vi "S71200_PLC_2.vi"(11 "Simulazione":bool) -> ()   [LabVIEW 2019]
uses:
  Uscite PLC 2.ctl
  controls/statoAO_plc_2.ctl
  StatoDO_PLC_2.ctl
  STATO PLC 2.ctl
  TypeDef_PLC_Q.ctl
  TypeDef/DEVICE NAME.ctl
  STATO PLC 1.ctl
  Uscite PLC 1.ctl
  controls/statoAO_plc_1.ctl
  StatoDO_PLC_1.ctl
  SIEMENS/S7Com_Source/S7Com_RW_CMD.ctl
  SIEMENS/S7Com_Source/S7Com_Address_Area.ctl
  SIEMENS/S7Com_Source/S7Com_Start_Add.ctl
  SIEMENS/S7Com_Source/S7Com_Transport_Size.ctl
  SIEMENS/S7Com_Source/S7Com_Function.ctl
panel:
  in  "millisecond multiple":u32=100
  out "write ao":errorcluster
  out "initialize":errorcluster
  in  "Tab Control":enum32{"PLC", "MERKER ", "DATABLOCK", "FGD"}(tab)
  out "STATO PLC":T1
  in  "write":bool
  in  "USCITE PLC":T2
  out "IP":string
  out "Simulazione 2":bool
  out "# elements in queue":i32
  out "DESC SCRITTURE MERKER WORD (AO)":string[][](array[string])
  out "Array WORD out":dbl[](array[numeric])
  out "DESC LETTURE MERKER WORD (AI)":string[][](array[string])
  out "MW read":dbl[](array[numeric])
  out "DESC SCRITTURE MERKER BIT (DO)":string[][](array[string])
  out "stato uscite DO":bool[](array[boolean])
  out "DESC LETTURE MERKER BIT (DI)":string[][](array[string])
  out "MBit read":bool[](array[boolean])
  out "DESC SCRITTURE MERKER REAK (AO)":string[][](array[string])
  out "DESC LETTURE MERKER REAL (AI)":string[][](array[string])
  out "Array M REAL out":dbl[](array[numeric])
  out "M Real":dbl[](array[numeric]) format="%.5f"
  out "DESC SCRITTURE DB BIT (DO)":string[][](array[string])
  out "DESC LETTURE DB BIT (DI)":string[][](array[string])
  out "DESC SCRITTURE DB WORD (AO)":string[][](array[string])
  out "DESC LETTURE DB WORD (AI)":string[][](array[string])
  out "DESC LETTURE DB REAL (AI)":string[][](array[string])
  out "DESC SCRITTURE DB REAL (AO)":string[][](array[string])
  out "DB WORD":dbl[](array[numeric])
  out "DB REAL":dbl[](array[numeric]) format="%.6f"
  out "Array DB bit":bool[](array[boolean])
  out "Array DB W out":dbl[](array[numeric])
  out "Array DB REAL out":dbl[](array[numeric]) format="%#.5f"
  out "DO (DATABLOCK)":bool[](array[boolean])
  out "M BIT SCRITTURE":cluster{"M":i16, "BIT":i16[]}[](array[cluster])
  out "M BIT LETTURE":cluster{"M":i16, "BIT":i16[]}[](array[cluster])
  out "MW SCRITTURE":T5(array[cluster])
  out "MW LETTURE":T5(array[cluster])
  out "M REAL LETTURE":cluster{"MD":i16, "Descrizione":string}[](array[cluster])
  out "M REAL SCRITTURE (AO)":cluster{"MD":i16, "Descrizione":string}[](array[cluster])
  out "DBW LETTURE":T6(array[cluster])
  out "DB REAL LETTURE":T7(array[cluster])
  out "DBW SCRITTURE":T6(array[cluster])
  out "DB REAL SCRITTURE":T7(array[cluster])
  out "DB BIT LETTURE":cluster{"DB":i16, "BIT":i16[], "DBoffset":i16}[](array[cluster])
  out "DB BIT SCRITTURE":cluster{"DB":i16, "BIT":i16[], "DBoffset":i16}[](array[cluster])
  out "Message":string
  out "write do":errorcluster
  out "read":errorcluster
  out "error out":errorcluster
  out "Numeric":i32
  out "Tread ms":u32
  in  "stop":bool
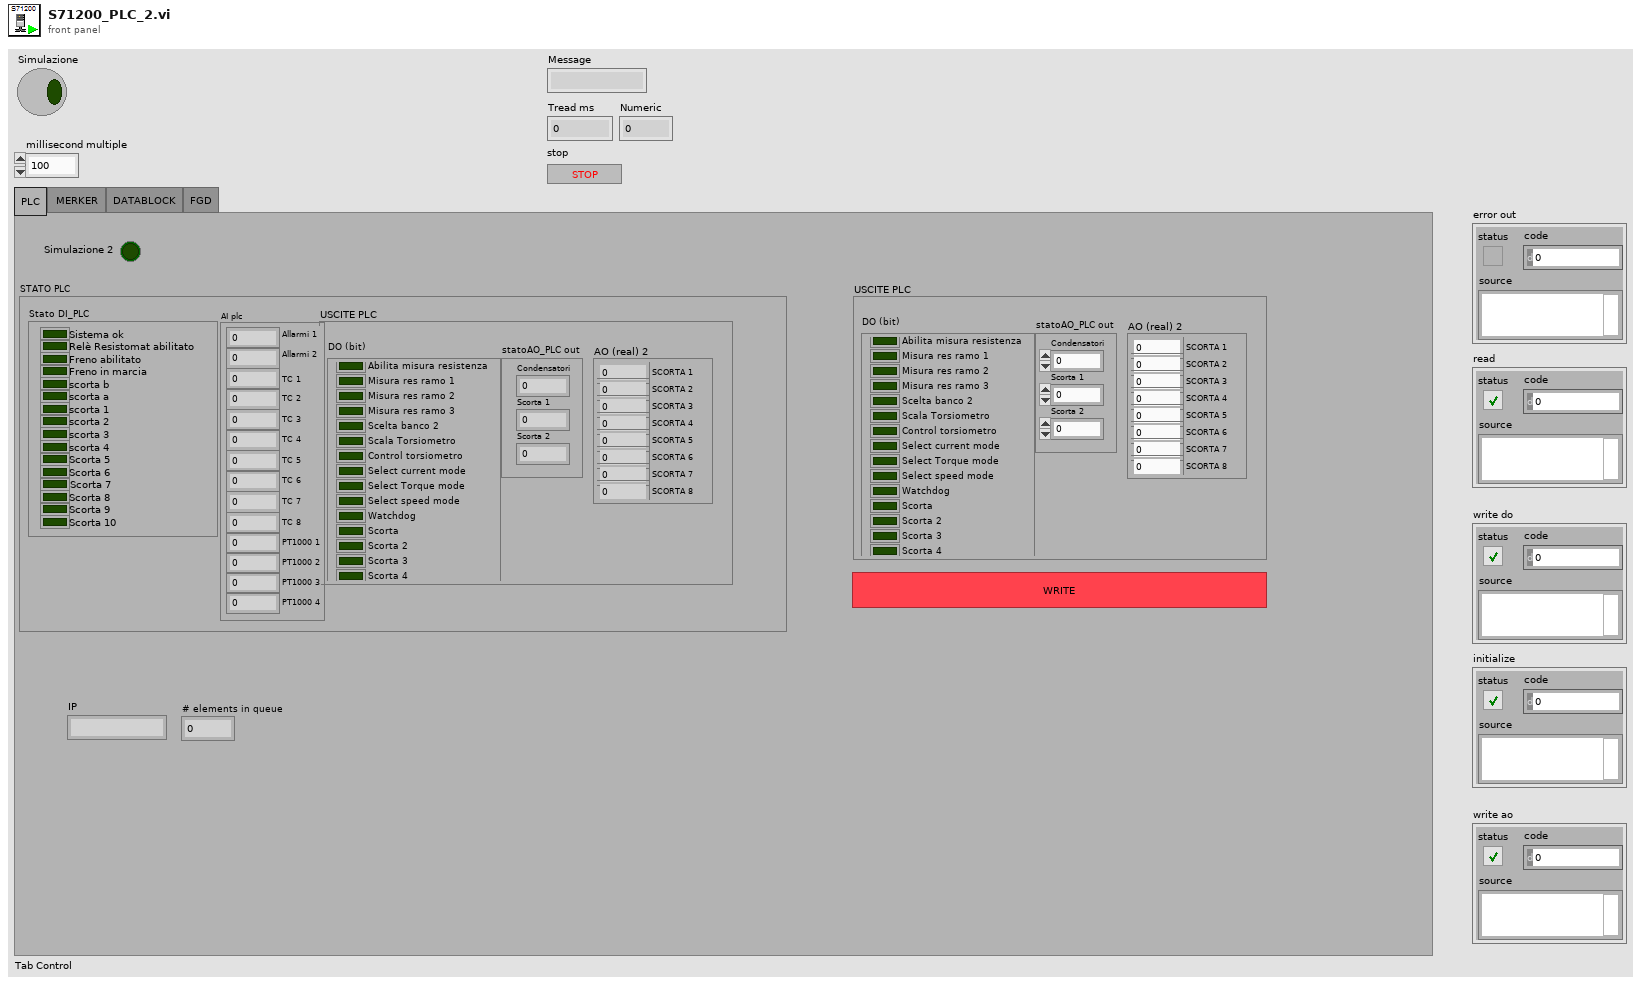
[diagram p1: front panel]
types:
  T1 = typedef "STATO PLC 2.ctl" = cluster{"USCITE PLC":T2, "Stato DI_PLC":cluster{"Sistema ok":bool, "Relè Resistomat abilitato":bool, "Freno abilitato":bool, "Freno in marcia":bool, "scorta b":bool, "scorta a":bool, "scorta 1":bool, "scorta 2":bool, "scorta 3":bool, "scorta 4":bool, "Scorta 5":bool, "Scorta 6":bool, "Scorta 7":bool, "Scorta 8":bool, "Scorta 9":bool, "Scorta 10":bool}, "AI plc":cluster{"Allarmi 1":dbl, "Allarmi 2":dbl, "TC 1":dbl, "TC 2":dbl, "TC 3":dbl, "TC 4":dbl, "TC 5":dbl, "TC 6":dbl, "TC 7":dbl, "TC 8":dbl, "PT1000 1":dbl, "PT1000 2":dbl, "PT1000 3":dbl, "PT1000 4":dbl}}
  T2 = typedef "Uscite PLC 2.ctl" = cluster{"AO (real) 2":cluster{"SCORTA 1":dbl, "SCORTA 2":dbl, "SCORTA 3":dbl, "SCORTA 4":dbl, "SCORTA 5":dbl, "SCORTA 6":dbl, "SCORTA 7":dbl, "SCORTA 8":dbl}, "statoAO_PLC out":T3, "DO (bit)":T4}
  T3 = typedef "statoAO_plc_2.ctl" = cluster{"Condensatori":dbl, "Scorta 1":dbl, "Scorta 2":dbl}
  T4 = typedef "StatoDO_PLC_2.ctl" = cluster{"Relè misura resistomat":bool, "Misura res ramo 1":bool, "Misura res ramo 2":bool, "Misura res ramo 3":bool, "Scelta banco 2":bool, "Scala Torsiometro":bool, "Ctrl torsiometro":bool, "Select current mode":bool, "Select Torque mode":bool, "Select speed mode":bool, "Watchdog":bool, "Scorta":bool, "Scorta 2":bool, "Scorta 3":bool, "Scorta 4":bool, "Scorta 5":bool, "Bench selection":bool, "External alarm":bool, "Enable external program":bool, "Reset allarmi":bool, "Start":bool, "Stop":bool, "Block":bool, "Scorta 6":bool}
  T5 = cluster{"MW":dbl, "Descrizione":string, "offset":dbl, "FS":dbl}[]
  T6 = cluster{"DB":i16, "DB offset":i16, "Descrizione":string, "offset":dbl, "FS":dbl}[]
  T7 = cluster{"DB":i16, "Descrizione":string, "DB offset":i16}[]
  T8 = typedef "TypeDef_PLC_Q.ctl" = cluster{"Message":string, "Data":variant}
  T9 = typedef "DEVICE NAME.ctl" = enum16{"WATTMETRO", "APLUS", "PLC BANCO 1", "PLC RACK", "PLC BANCO 2", "PS", "NI cDAQ", "RESISTOMAT"}
  T10 = typedef "S7Com_RW_CMD.ctl" = cluster{"Read Length":u16, "Data Block #":u16, "S7_Add_Area":T11, "Start Address":T12, "S7_Transport_Size":T13, "S7_Function":T14}
  T11 = typedef "S7Com_Address_Area.ctl" = u8
  T12 = typedef "S7Com_Start_Add.ctl" = u16
  T13 = typedef "S7Com_Transport_Size.ctl" = u8
  T14 = typedef "S7Com_Function.ctl" = u8
  T15 = cluster{cluster{string[][], cluster{"MW":dbl, "Descrizione":string, "offset":dbl, "FS":dbl}[]}, cluster{string[][], cluster{"MD":i16, "Descrizione":string}[]}, cluster{string[][], cluster{"MW":dbl, "Descrizione":string, "offset":dbl, "FS":dbl}[]}, cluster{string[][], cluster{"MD":i16, "Descrizione":string}[]}, cluster{string[][], cluster{"M":i16, "BIT":i16[]}[]}, cluster{string[][], cluster{"M":i16, "BIT":i16[]}[]}}
  T16 = cluster{cluster{string[][], cluster{"DB":i16, "DB offset":i16, "Descrizione":string, "offset":dbl, "FS":dbl}[]}, cluster{string[][], cluster{"DB":i16, "Descrizione":string, "DB offset":i16}[]}, cluster{string[][], cluster{"DB":i16, "DB offset":i16, "Descrizione":string, "offset":dbl, "FS":dbl}[]}, cluster{string[][], cluster{"DB":i16, "Descrizione":string, "DB offset":i16}[]}, cluster{string[][], cluster{"DB":i16, "BIT":i16[], "DBoffset":i16}[]}, cluster{string[][], cluster{"DB":i16, "BIT":i16[], "DBoffset":i16}[]}}
  T17 = cluster{string[][], cluster{"MW":dbl, "Descrizione":string, "offset":dbl, "FS":dbl}[]}
  T18 = cluster{string[][], cluster{"MD":i16, "Descrizione":string}[]}
  T19 = cluster{string[][], cluster{"M":i16, "BIT":i16[]}[]}
  T20 = cluster{string[][], cluster{"DB":i16, "DB offset":i16, "Descrizione":string, "offset":dbl, "FS":dbl}[]}
  T21 = cluster{string[][], cluster{"DB":i16, "Descrizione":string, "DB offset":i16}[]}
  T22 = cluster{string[][], cluster{"DB":i16, "BIT":i16[], "DBoffset":i16}[]}
  T23 = typedef "STATO PLC 1.ctl" = cluster{"USCITE PLC":T24, "Stato DI_PLC":cluster{"Sistema OK":bool, "Rotore bloccato":bool, "Scorta 1":bool, "Prova diretto inverter":bool, "Prova con filtro LC":bool, "Teleruttore WT abilitato":bool, "Alim sinus penta abilitato":bool, "Alim sinus penta in marcia":bool, "Freno abilitato":bool, "Freno in marcia":bool, "Senso rotazione freno":bool, "Potenza abilitata":bool, "Scorta 3":bool, "Scorta 4":bool, "scorta 5":bool, "scorta 6":bool}, "AI plc":cluster{"Allarmi 1":dbl, "Allarmi 2":dbl, "Scorta 1":dbl, "Scorta 2":dbl, "RPM mot prova":dbl, "I mot prova":dbl, "RPM freno":dbl, "I freno":dbl, "Scorta 3":dbl, "Scorta 4":dbl}}
  T24 = typedef "Uscite PLC 1.ctl" = cluster{"AO (real) 2":cluster{"SCORTA 1":dbl, "SCORTA 2":dbl, "SCORTA 3":dbl, "SCORTA 4":dbl, "SCORTA 5":dbl, "SCORTA 6":dbl, "SCORTA 7":dbl, "SCORTA 8":dbl}, "statoAO_PLC out":T25, "DO (bit)":T26}
  T25 = typedef "statoAO_plc_1.ctl" = cluster{"Rif Lim coppia freno [%]":dbl, "Rif rpm freno [%]":dbl, "Rif coppia freno [%]":dbl, "Rif V alimentatore [%]":dbl, "Rif F alimentatore [%]":dbl}
  T26 = typedef "StatoDO_PLC_1.ctl" = cluster{"Scelta banco 1":bool, "Set dati motore freno 2":bool, "Diretto inverter":bool, "Filtro LC":bool, "Marcia ALIM (1s)":bool, "Marcia FRENO (1s)":bool, "Stop AFE (1s)":bool, "Stop freno (1s)":bool, "Reset allarmi":bool, "Watchdog":bool, "Senso rotazione":bool, "Abilita collaudo (1s)":bool, "Disabilita collaudo (1s)":bool, "Abilitazione ALIM":bool, "Abilitazione FRENO":bool, "Teleruttore WT":bool, "Senso rot motore prova":bool, "Scorta 7":bool, "Scorta 8":bool, "Scorta 9":bool, "Scorta 10":bool, "Scorta 11":bool, "Scorta 12":bool, "Scorta 13":bool}
  T27 = cluster{"SCORTA 1":dbl, "SCORTA 2":dbl, "SCORTA 3":dbl, "SCORTA 4":dbl, "SCORTA 5":dbl, "SCORTA 6":dbl, "SCORTA 7":dbl, "SCORTA 8":dbl}
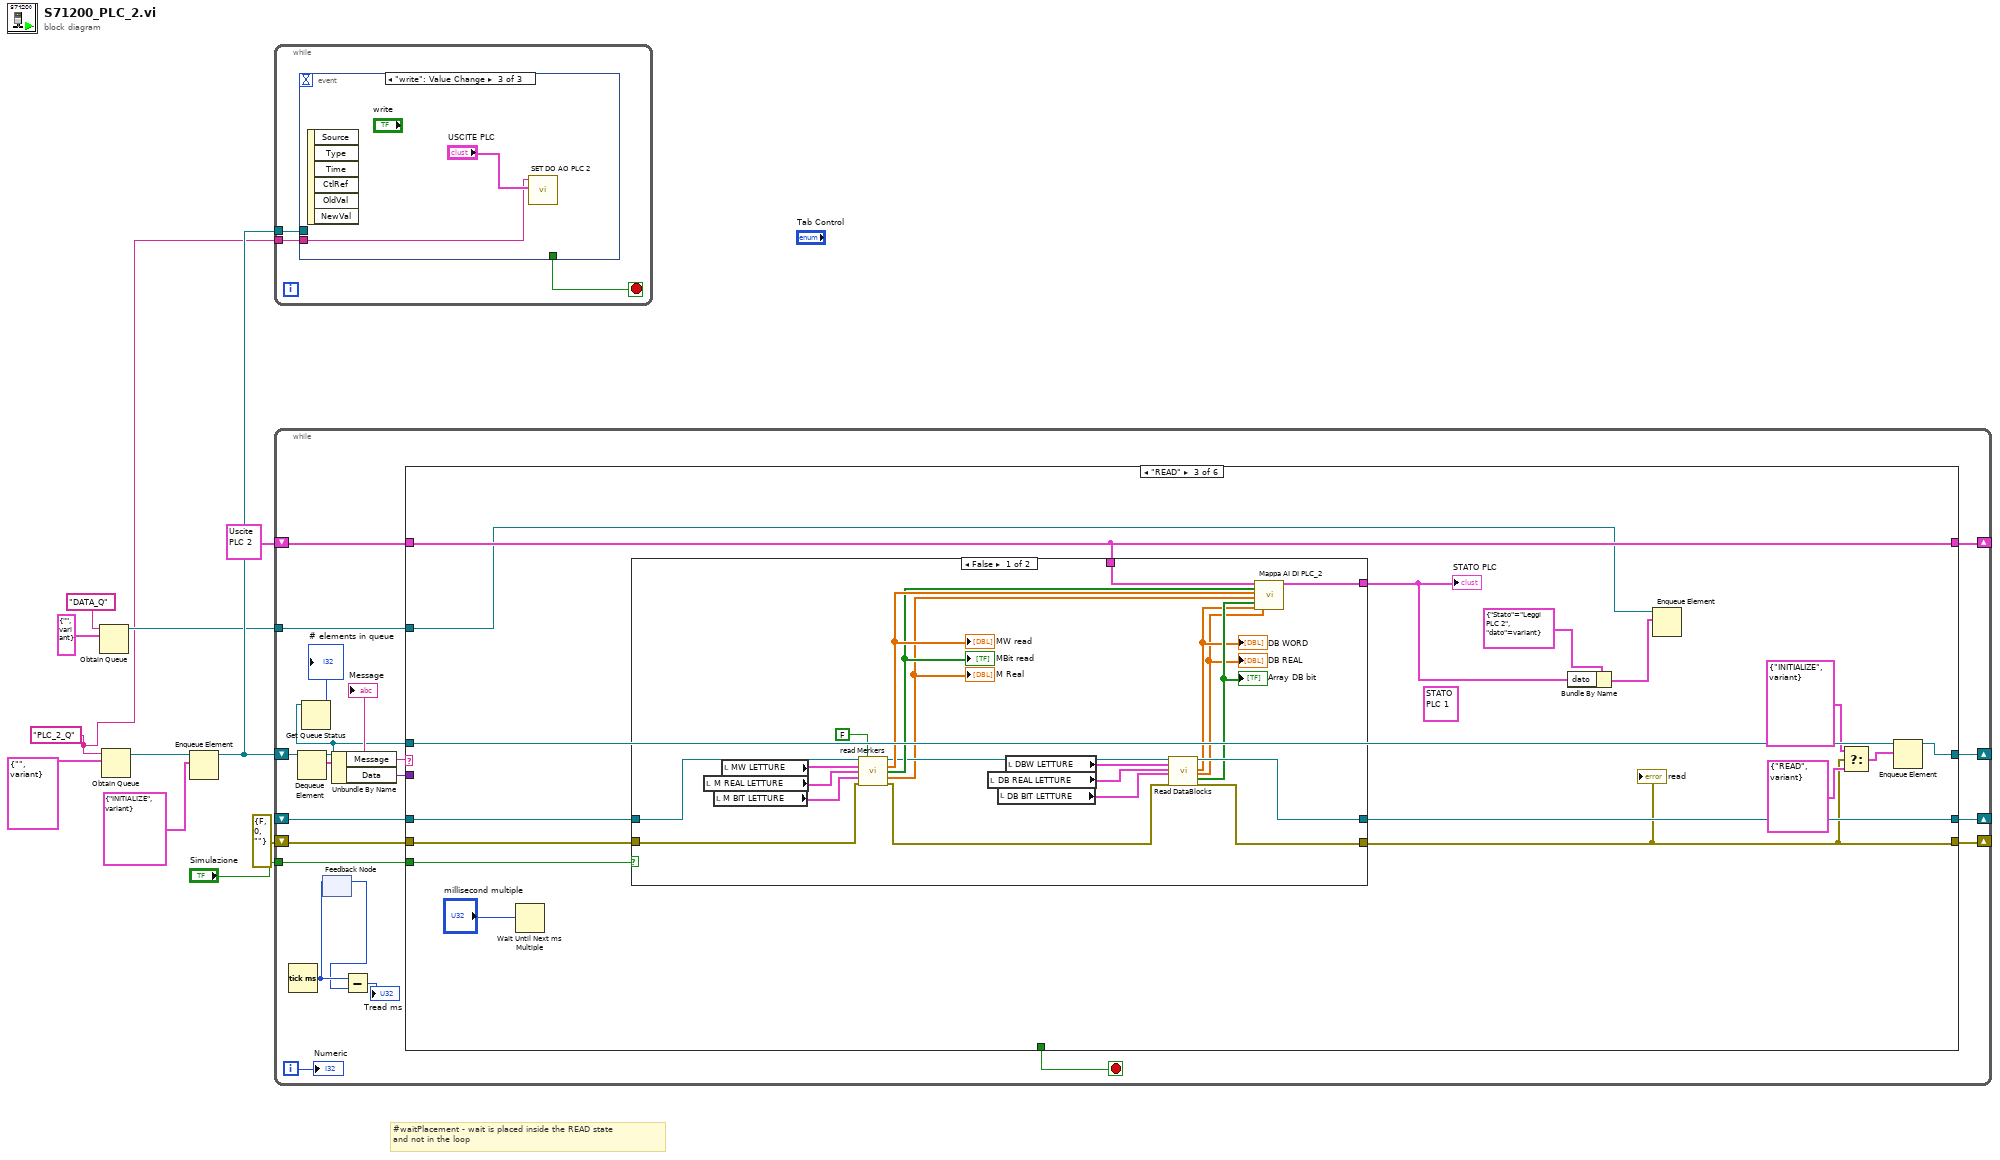
[diagram p0: block diagram]
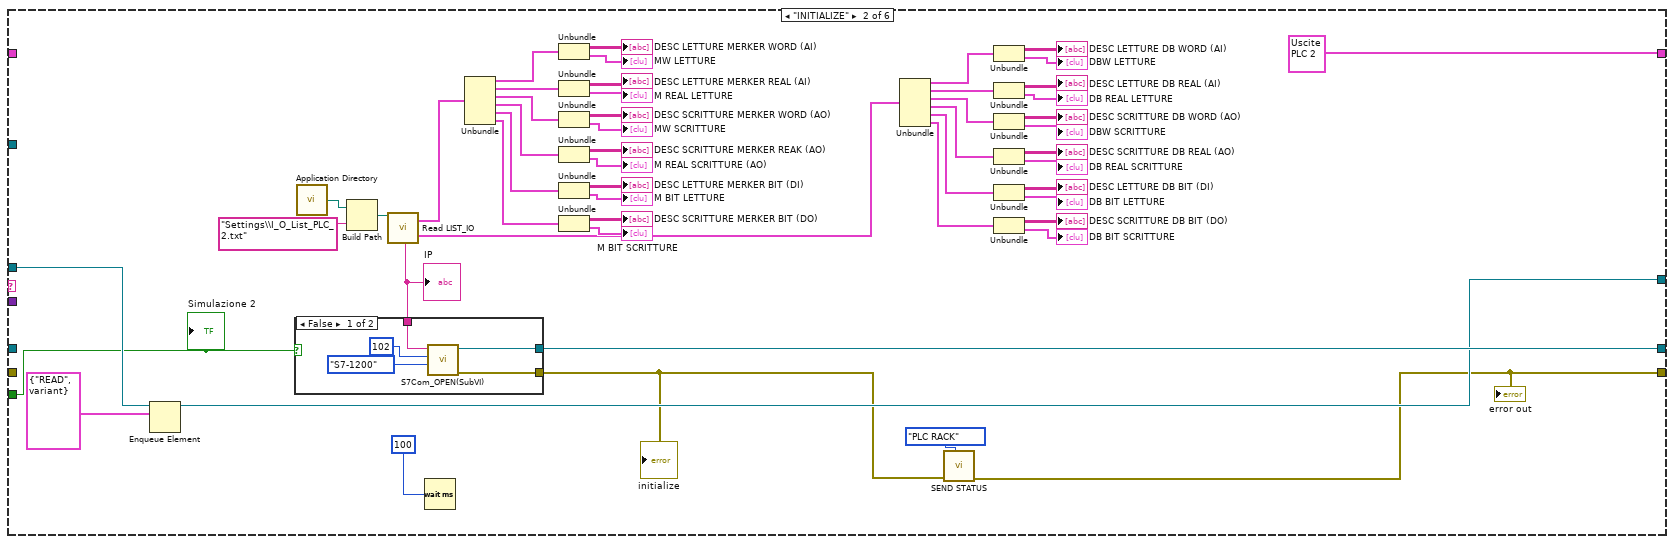
[diagram p3: hidden frame]
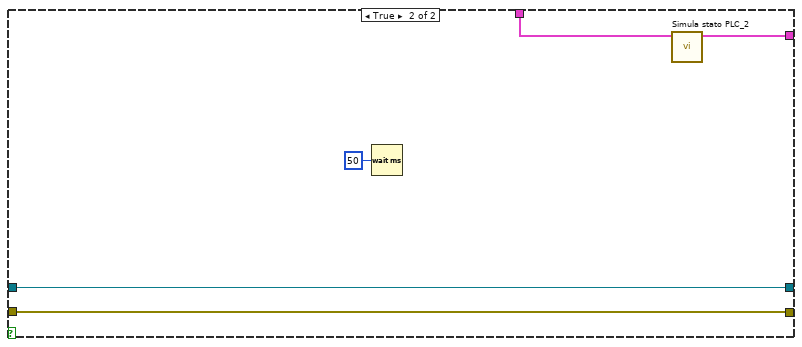
[diagram p5: hidden frame]
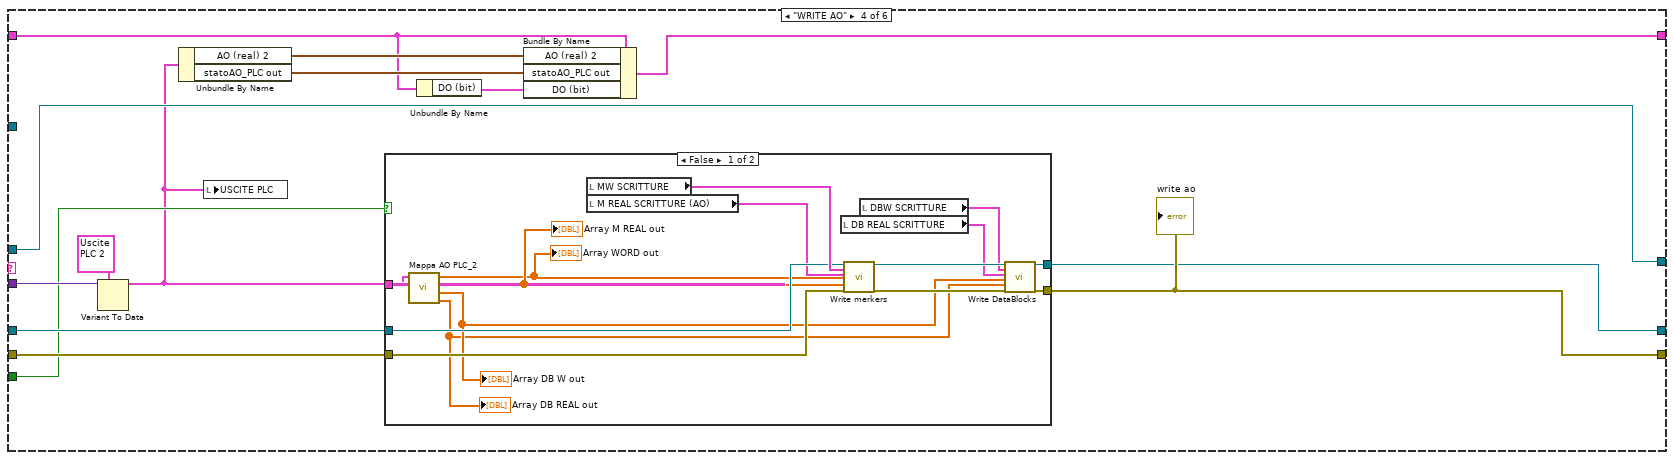
[diagram p6: hidden frame]
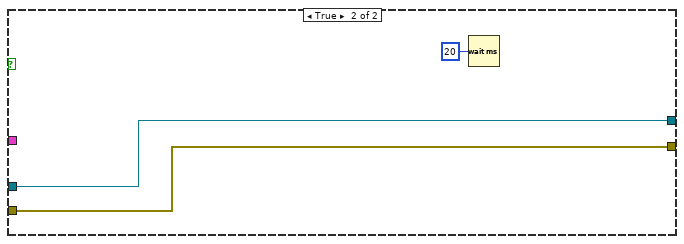
[diagram p7: hidden frame]
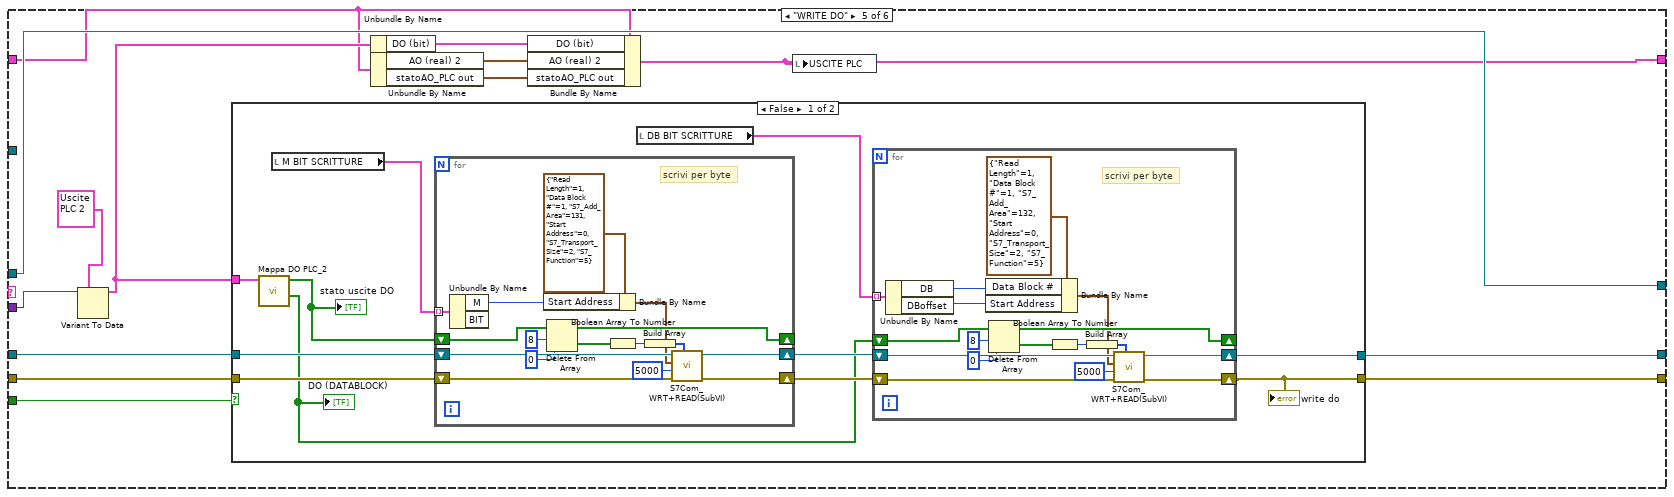
[diagram p8: hidden frame]
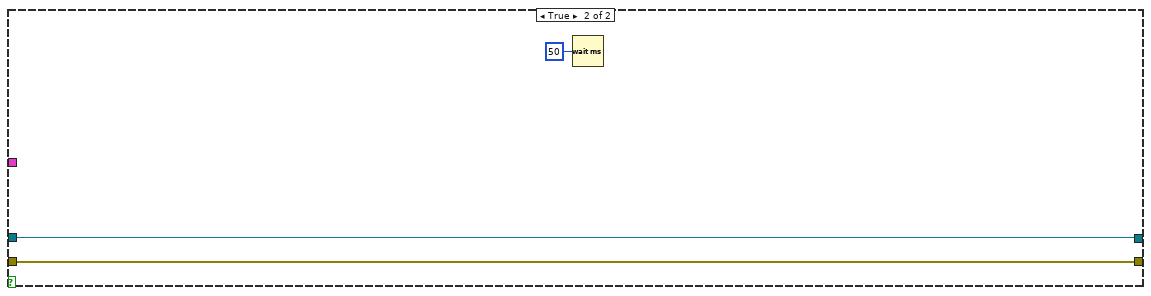
[diagram p9: hidden frame]
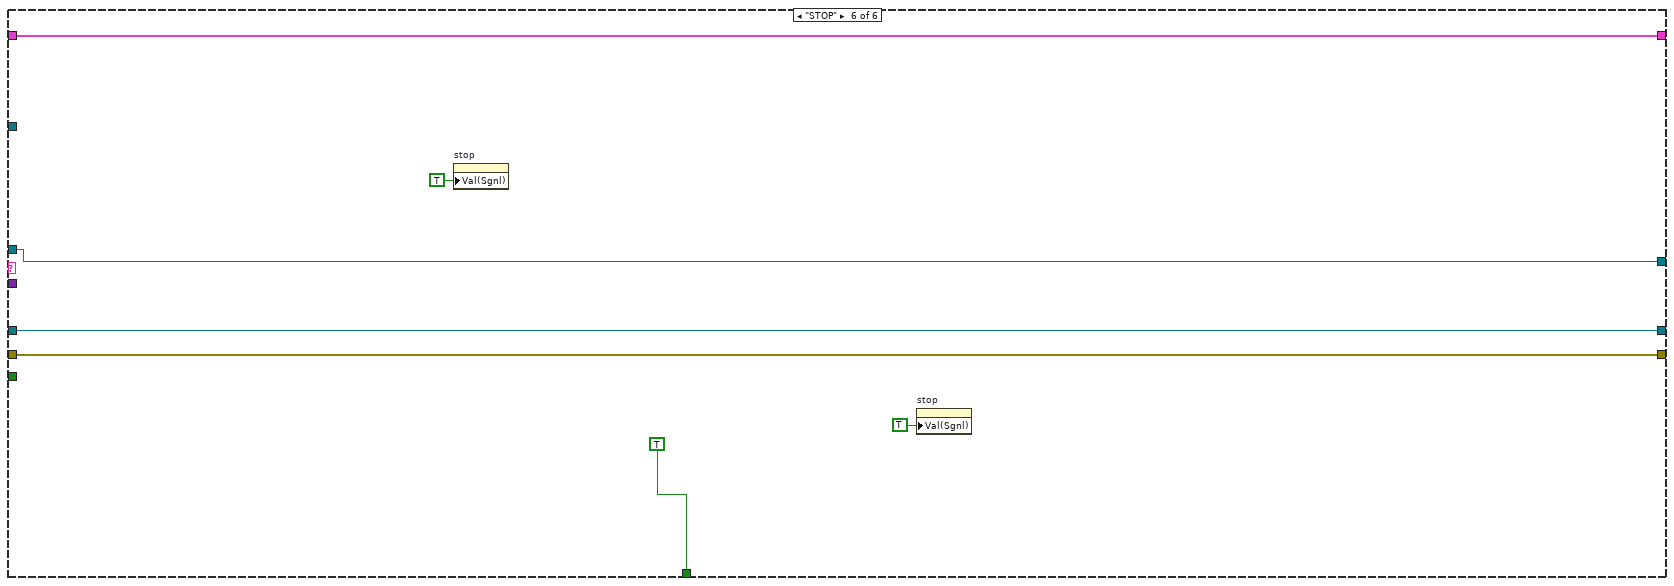
[diagram p10: hidden frame]
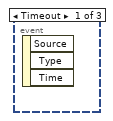
[diagram p11: hidden frame]
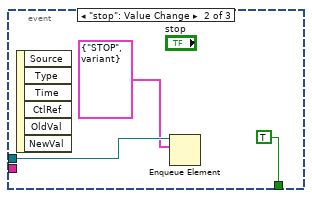
[diagram p12: hidden frame]
diagram:
  w1 = "PLC_2_Q" ("name (unnamed)")
  # "#waitPlacement - wait is placed inside the READ state \nand not in the loop"
  n1 = Obtain Queue(name (unnamed)="DATA_Q", element data type=cluster{"Stato":string, "dato":variant} {"Stato"="", "dato"=variant} ("Cluster")) -> (queue out=w3:refnum<queue>)  [unwired: 3 in, 2 out]
  n2 = Obtain Queue(name (unnamed)=w1, element data type=T8 {"Message"="", "Data"=variant}) -> (queue out=w10:refnum<queue>)  [unwired: 3 in, 2 out]
  n3 = Enqueue Element(queue=w10, element=T8 {"Message"="INITIALIZE", "Data"=variant}) -> (queue out=w9:refnum<queue>)  [unwired: 2 in, 2 out]
  n4 = while {
    tunnel: w9 -> [w13]
    tunnel: w1 -> [w12]
    stop <- w14 stop-if-true
    n5 = event shown="[2] \"write\": Value Change" {
      selector: _ -> [_ _ _]
      dyn-events: _ -> [_ _ _]
      timeout: _ -> [_ _ _]
      tunnel: [_ TRUE _] -> w14
      tunnel: w13 -> [_ w16 _]
      tunnel: w12 -> [_ _ w18]
      event Timeout {
        n6 = event-data() -> ()  [unwired: 1 in, 3 out]
      }
      event "stop": Value Change {
        n7 = event-data() -> ()  [unwired: 1 in, 6 out]
        n8 = Enqueue Element(queue=w16, element=cluster{"Message":string, "Data":variant} {"Message"="STOP", "Data"=variant}) -> ()  [unwired: 2 in, 3 out]
      }
      event "write": Value Change {
        n9 = event-data() -> ()  [unwired: 1 in, 6 out]
        n10 = call "SET DO AO PLC 2.vi"("USCITE PLC"="USCITE PLC", "Q"=w18) -> ()  [unwired: 10 in]
      }
    }
  }
  n11 = while {
    shift-right: [w30] -> _
    shift-left: w9 -> [w36]
    shift-right: [w35] -> _
    shift-left: _ -> [w33]
    shift-right: [w34] -> _
    shift-left: errorcluster {"status"=FALSE, "code"=0, "source"=""} ("error out") -> [w32]
    shift-right: [w25] -> _
    shift-left: T2 {"AO (real) 2"={"SCORTA 1"=0.0, "SCORTA 2"=0.0, "SCORTA 3"=0.0, "SCORTA 4"=0.0, "SCORTA 5"=0.0, "SCORTA 6"=0.0, "SCORTA 7"=0.0, "SCORTA 8"=0.0}, "statoAO_PLC out"={"Condensatori"=0.0, "Scorta 1"=0.0, "Scorta 2"=0.0}, "DO (bit)"={"Relè misura resistomat"=FALSE, "Misura res ramo 1"=FALSE, "Misura res ramo 2"=FALSE, "Misura res ramo 3"=FALSE, "Scelta banco 2"=FALSE, "Scala Torsiometro"=FALSE, "Ctrl torsiometro"=FALSE, "Select current mode"=FALSE, "Select Torque mode"=FALSE, "Select speed mode"=FALSE, "Watchdog"=FALSE, "Scorta"=FALSE, "Scorta 2"=FALSE, "Scorta 3"=FALSE, "Scorta 4"=FALSE, "Scorta 5"=FALSE, "Bench selection"=FALSE, "External alarm"=FALSE, "Enable external program"=FALSE, "Reset allarmi"=FALSE, "Start"=FALSE, "Stop"=FALSE, "Block"=FALSE, "Scorta 6"=FALSE}} ("USCITE PLC") -> [w24]
    tunnel: "Simulazione" -> [w23]
    tunnel: w3 -> [w22]
    i -> [w26]
    stop <- w31 stop-if-true
    n12 = Tick Count (ms)() -> (millisecond timer value=w29:u32)
    n13 = Dequeue Element(queue=w36) -> (queue out=w21:refnum<queue>, element=w39:T8)  [unwired: 2 in, 2 out]
    n14 = Get Queue Status(queue=w21) -> (# elements in queue=→"# elements in queue":i32)  [unwired: 2 in, 7 out]
    n15 = feedback-in #1(w29) -> ()
    n16 = feedback #1() -> (w28:u32)  [unwired: 1 in]
    n17 = Unbundle By Name(w39) -> ("Message"=w38:string, "Data"=w37:variant)
    "Message" <- w38
    n18 = Subtract(x=w29, y=w28) -> (x-y=→"Tread ms":u32)
    n19 = case shown="\"READ\"" w38 {
      tunnel: w37 -> [_ _ _ w152 w185 _]
      tunnel: [w43 w95 w110 w150 w184 w241] -> w35
      tunnel: [w42 w45 w101 w151 w183 w240] -> w34
      tunnel: w33 -> [w43 _ w116 w156 w188 w241]
      tunnel: w32 -> [w42 _ w115 w155 w187 w240]
      tunnel: [_ _ _ _ _ TRUE] -> w31
      tunnel: w21 -> [w41 w90 w114 w154 w186 w239]
      tunnel: [w41 w89 w113 w154 w186 w239] -> w30
      tunnel: [w40 T2 {"AO (real) 2"={"SCORTA 1"=0.0, "SCORTA 2"=0.0, "SCORTA 3"=0.0, "SCORTA 4"=0.0, "SCORTA 5"=0.0, "SCORTA 6"=0.0, "SCORTA 7"=0.0, "SCORTA 8"=0.0}, "statoAO_PLC out"={"Condensatori"=0.0, "Scorta 1"=0.0, "Scorta 2"=0.0}, "DO (bit)"={"Relè misura resistomat"=FALSE, "Misura res ramo 1"=FALSE, "Misura res ramo 2"=FALSE, "Misura res ramo 3"=FALSE, "Scelta banco 2"=FALSE, "Scala Torsiometro"=FALSE, "Ctrl torsiometro"=FALSE, "Select current mode"=FALSE, "Select Torque mode"=FALSE, "Select speed mode"=FALSE, "Watchdog"=FALSE, "Scorta"=FALSE, "Scorta 2"=FALSE, "Scorta 3"=FALSE, "Scorta 4"=FALSE, "Scorta 5"=FALSE, "Bench selection"=FALSE, "External alarm"=FALSE, "Enable external program"=FALSE, "Reset allarmi"=FALSE, "Start"=FALSE, "Stop"=FALSE, "Block"=FALSE, "Scorta 6"=FALSE}} ("USCITE PLC") w111 w147 w179 w238] -> w25
      tunnel: w24 -> [w40 _ w111 w144 w178 w238]
      tunnel: w23 -> [_ w48 w109 w149 w182 _]
      tunnel: w22 -> [_ _ w105 _ _ _]
      frame "False", Default {
      }
      frame "INITIALIZE" {
        n20 = Enqueue Element(queue=w90, element=T8 {"Message"="READ", "Data"=variant}) -> (queue out=w89:refnum<queue>)  [unwired: 2 in, 2 out]
        n21 = call <vilib>:"Application Directory.vi"() -> ("Application Directory"=w92:path)
        n22 = Build Path(base path=w92, name or relative path="Settings\\I_O_List_PLC_2.txt") -> (appended path=w91:path)
        n23 = call "Read LIST_IO.vi"("file (use dialog)"=w91) -> ("IP"=w94:string, "MERKER"=w87:T15, "DATABLOCK"=w56:T16)  [unwired: 16 in]
        "IP" <- w94
        n24 = case shown="False" w48 {
          tunnel: [w98 _] -> w95
          tunnel: [w97 _] -> w46
          tunnel: w94 -> [w96 _]
          frame False {
            n25 = call "S7Com_OPEN(SubVI).vi"("PLC type"=enum16{"S7-300", "S7-1200"}."S7-1200", "remote port"=u16 102, "remote address"=w96) -> ("error out"=w97:errorcluster, "connection ID out"=w98:refnum<k5>)  [unwired: 4 in, 3 out]
          }
          frame True {
          }
        }
        "initialize" <- w46
        n26 = Wait (ms)(milliseconds to wait=u32 100) -> ()  [unwired: 1 out]
        n27 = Unbundle(w87) -> (w86:T17, w83:T18, w82:T17, w79:T18, w78:T19, w75:T19)
        n28 = Unbundle(w86) -> (→"DESC LETTURE MERKER WORD (AI)":string[][], →"MW LETTURE":T5)
        n29 = Unbundle(w83) -> (→"DESC LETTURE MERKER REAL (AI)":string[][], →"M REAL LETTURE":cluster{"MD":i16, "Descrizione":string}[])
        n30 = Unbundle(w82) -> (→"DESC SCRITTURE MERKER WORD (AO)":string[][], →"MW SCRITTURE":T5)
        n31 = Unbundle(w79) -> (→"DESC SCRITTURE MERKER REAK (AO)":string[][], →"M REAL SCRITTURE (AO)":cluster{"MD":i16, "Descrizione":string}[])
        n32 = Unbundle(w78) -> (→"DESC LETTURE MERKER BIT (DI)":string[][], →"M BIT LETTURE":cluster{"M":i16, "BIT":i16[]}[])
        n33 = Unbundle(w75) -> (→"DESC SCRITTURE MERKER BIT (DO)":string[][], →"M BIT SCRITTURE":cluster{"M":i16, "BIT":i16[]}[])
        n34 = Unbundle(w56) -> (w57:T20, w59:T21, w60:T20, w62:T21, w63:T22, w65:T22)
        n35 = call "SEND STATUS.vi"("ELEMENT"=DEVICE_NAME."PLC RACK", "error in (no error)"=w46) -> ("error out"=w45:errorcluster)  [unwired: 9 in]
        "error out" <- w45
        n36 = Unbundle(w57) -> (→"DESC LETTURE DB WORD (AI)":string[][], →"DBW LETTURE":T6)
        n37 = Unbundle(w59) -> (→"DESC LETTURE DB REAL (AI)":string[][], →"DB REAL LETTURE":T7)
        n38 = Unbundle(w60) -> (→"DESC SCRITTURE DB WORD (AO)":string[][], →"DBW SCRITTURE":T6)
        n39 = Unbundle(w62) -> (→"DESC SCRITTURE DB REAL (AO)":string[][], →"DB REAL SCRITTURE":T7)
        n40 = Unbundle(w63) -> (→"DESC LETTURE DB BIT (DI)":string[][], →"DB BIT LETTURE":cluster{"DB":i16, "BIT":i16[], "DBoffset":i16}[])
        n41 = Unbundle(w65) -> (→"DESC SCRITTURE DB BIT (DO)":string[][], →"DB BIT SCRITTURE":cluster{"DB":i16, "BIT":i16[], "DBoffset":i16}[])
        "Simulazione 2" <- w48
      }
      frame "READ" {
        (unwired) T23 {"USCITE PLC"={"AO (real) 2"={"SCORTA 1"=0.0, "SCORTA 2"=0.0, "SCORTA 3"=0.0, "SCORTA 4"=0.0, "SCORTA 5"=0.0, "SCORTA 6"=0.0, "SCORTA 7"=0.0, "SCORTA 8"=0.0}, "statoAO_PLC out"={"Rif Lim coppia freno [%]"=0.0, "Rif rpm freno [%]"=0.0, "Rif coppia freno [%]"=0.0, "Rif V alimentatore [%]"=0.0, "Rif F alimentatore [%]"=0.0}, "DO (bit)"={"Scelta banco 1"=FALSE, "Set dati motore freno 2"=FALSE, "Diretto inverter"=FALSE, "Filtro LC"=FALSE, "Marcia ALIM (1s)"=FALSE, "Marcia FRENO (1s)"=FALSE, "Stop AFE (1s)"=FALSE, "Stop freno (1s)"=FALSE, "Reset allarmi"=FALSE, "Watchdog"=FALSE, "Senso rotazione"=FALSE, "Abilita collaudo (1s)"=FALSE, "Disabilita collaudo (1s)"=FALSE, "Abilitazione ALIM"=FALSE, "Abilitazione FRENO"=FALSE, "Teleruttore WT"=FALSE, "Senso rot motore prova"=FALSE, "Scorta 7"=FALSE, "Scorta 8"=FALSE, "Scorta 9"=FALSE, "Scorta 10"=FALSE, "Scorta 11"=FALSE, "Scorta 12"=FALSE, "Scorta 13"=FALSE}}, "Stato DI_PLC"={"Sistema OK"=FALSE, "Rotore bloccato"=TRUE, "Scorta 1"=FALSE, "Prova diretto inverter"=FALSE, "Prova con filtro LC"=FALSE, "Teleruttore WT abilitato"=FALSE, "Alim sinus penta abilitato"=FALSE, "Alim sinus penta in marcia"=FALSE, "Freno abilitato"=FALSE, "Freno in marcia"=FALSE, "Senso rotazione freno"=FALSE, "Potenza abilitata"=FALSE, "Scorta 3"=FALSE, "Scorta 4"=FALSE, "scorta 5"=FALSE, "scorta 6"=FALSE}, "AI plc"={"Allarmi 1"=0.0, "Allarmi 2"=0.0, "Scorta 1"=0.0, "Scorta 2"=0.0, "RPM mot prova"=0.0, "I mot prova"=0.0, "RPM freno"=0.0, "I freno"=0.0, "Scorta 3"=0.0, "Scorta 4"=0.0}} ("STATO PLC")
        n42 = Wait Until Next ms Multiple(millisecond multiple="millisecond multiple") -> ()  [unwired: 1 out]
        n43 = case shown="False" w109 {
          tunnel: w116 -> [w136 w142]
          tunnel: w115 -> [w135 w141]
          tunnel: w111 -> [w133 w140]
          tunnel: [w132 w139] -> w102
          tunnel: [w127 w142] -> w110
          tunnel: [w125 w141] -> w101
          frame False {
            n44 = local read "M REAL LETTURE"() -> (w131:cluster{"MD":i16, "Descrizione":string}[])
            n45 = local read "M BIT LETTURE"() -> (w130:cluster{"M":i16, "BIT":i16[]}[])
            n46 = local read "MW LETTURE"() -> (w137:T5)
            n47 = call "read Merkers.vi"("TCP Network Connection in"=w136, "U16?"=FALSE, "MW LETTURE"=w137, "M REAL LETTURE"=w131, "M BIT LETTURE"=w130, "error in (no error)"=w135) -> ("TCP Network Connection out"=w128:refnum<k5>, "MW"=w134:dbl[], "Array M bit"=w129:bool[], "M Real"=w121:dbl[], "error out"=w126:errorcluster)  [unwired: 5 in]
            "MW read" <- w134
            "MBit read" <- w129
            "M Real" <- w121
            n48 = local read "DB REAL LETTURE"() -> (w123:T7)
            n49 = local read "DB BIT LETTURE"() -> (w122:cluster{"DB":i16, "BIT":i16[], "DBoffset":i16}[])
            n50 = local read "DBW LETTURE"() -> (w124:T6)
            n51 = call "Read DataBlocks.vi"("TCP Network Connection in"=w128, "DBW LETTURE"=w124, "DB REAL LETTURE"=w123, "DB BIT LETTURE"=w122, "error in (no error)"=w126) -> ("TCP Network Connection out"=w127:refnum<k5>, "DB WORD"=w119:dbl[], "DB REAL"=w118:dbl[], "Array DB bit"=w120:bool[], "error out"=w125:errorcluster)  [unwired: 10 in]
            "DB WORD" <- w119
            "DB REAL" <- w118
            "Array DB bit" <- w120
            n52 = call "Mappa AI DI PLC_2.vi"("USCITE PLC"=w133, "MBit read"=w129, "MW read"=w134, "M real read"=w121, "Array DB bit"=w120, "DB WORD"=w119, "DB REAL"=w118) -> ("STATO PLC"=w132:T1)  [unwired: 12 in]
          }
          frame True {
            n53 = Wait (ms)(milliseconds to wait=u32 50) -> ()  [unwired: 1 out]
            n54 = call "Simula stato PLC_2.vi"("USCITE PLC"=w140) -> ("STATO PLC"=w139:T1)  [unwired: 10 in]
          }
        }
        "read" <- w101
        "STATO PLC" <- w102
        n55 = Bundle By Name(cluster=cluster{"Stato":string, "dato":variant} {"Stato"="Leggi PLC 2", "dato"=variant} ("Cluster"), "dato"=w102) -> (w103:cluster{"Stato":string, "dato":variant})
        n56 = Enqueue Element(queue=w105, element=w103) -> ()  [unwired: 2 in, 3 out]
        n57 = Select(t=T8 {"Message"="INITIALIZE", "Data"=variant}, s=w101, f=T8 {"Message"="READ", "Data"=variant}) -> (s? t:f=w107:T8)
        n58 = Enqueue Element(queue=w114, element=w107) -> (queue out=w113:refnum<queue>)  [unwired: 2 in, 2 out]
      }
      frame "WRITE AO" {
        n59 = Variant To Data(type=T2 {"AO (real) 2"={"SCORTA 1"=0.0, "SCORTA 2"=0.0, "SCORTA 3"=0.0, "SCORTA 4"=0.0, "SCORTA 5"=0.0, "SCORTA 6"=0.0, "SCORTA 7"=0.0, "SCORTA 8"=0.0}, "statoAO_PLC out"={"Condensatori"=nan, "Scorta 1"=nan, "Scorta 2"=0.0}, "DO (bit)"={"Relè misura resistomat"=FALSE, "Misura res ramo 1"=FALSE, "Misura res ramo 2"=FALSE, "Misura res ramo 3"=FALSE, "Scelta banco 2"=FALSE, "Scala Torsiometro"=FALSE, "Ctrl torsiometro"=FALSE, "Select current mode"=FALSE, "Select Torque mode"=FALSE, "Select speed mode"=FALSE, "Watchdog"=FALSE, "Scorta"=FALSE, "Scorta 2"=FALSE, "Scorta 3"=FALSE, "Scorta 4"=FALSE, "Scorta 5"=FALSE, "Bench selection"=FALSE, "External alarm"=FALSE, "Enable external program"=FALSE, "Reset allarmi"=FALSE, "Start"=FALSE, "Stop"=FALSE, "Block"=FALSE, "Scorta 6"=FALSE}} ("USCITE PLC"), Variant=w152) -> (data=w148:T2)  [unwired: 1 in, 1 out]
        n60 = Unbundle By Name(w148) -> ("AO (real) 2"=w146:T27, "statoAO_PLC out"=w145:T3)
        n61 = local write "USCITE PLC"(w148) -> ()
        n62 = case shown="False" w149 {
          tunnel: w156 -> [w170 w174]
          tunnel: w155 -> [w169 w173]
          tunnel: w148 -> [w157 _]
          tunnel: [w164 w173] -> w151
          tunnel: [w163 w174] -> w150
          frame False {
            n63 = call "Mappa AO PLC_2.vi"("USCITE PLC 2"=w157) -> ("Array DB REAL out"=w159:dbl[], "Array DB W out"=w160:dbl[], "Array M REAL out"=w167:dbl[], "Array M WORD out"=w158:dbl[])  [unwired: 7 in]
            "Array WORD out" <- w158
            "Array M REAL out" <- w167
            "Array DB W out" <- w160
            "Array DB REAL out" <- w159
            n64 = local read "MW SCRITTURE"() -> (w171:T5)
            n65 = local read "M REAL SCRITTURE (AO)"() -> (w168:cluster{"MD":i16, "Descrizione":string}[])
            n66 = local read "DB REAL SCRITTURE"() -> (w161:T7)
            n67 = call "Write merkers.vi"("TCP Network Connection in"=w170, "MW SCRITTURE"=w171, "M REAL SCRITTURE (AO)"=w168, "AO (word)"=w158, "AO (real) in"=w167, "error in (no error)"=w169) -> ("TCP Network Connection out"=w166:refnum<k5>, "error out"=w165:errorcluster)  [unwired: 12 in]
            n68 = local read "DBW SCRITTURE"() -> (w162:T6)
            n69 = call "Write DataBlocks.vi"("connection ID out"=w166, "DBW SCRITTURE"=w162, "DB REAL SCRITTURE"=w161, "DB AO (word)"=w160, "DB AO (real)"=w159, "error out"=w165) -> ("connection ID out"=w163:refnum<k5>, "error out"=w164:errorcluster)  [unwired: 12 in]
          }
          frame True {
            n70 = Wait (ms)(milliseconds to wait=u32 20) -> ()  [unwired: 1 out]
          }
        }
        "write ao" <- w151
        n71 = Unbundle By Name(w144) -> ("DO (bit)"=w143:T4)
        n72 = Bundle By Name(cluster=w144, "AO (real) 2"=w146, "statoAO_PLC out"=w145, "DO (bit)"=w143) -> (w147:T2)
      }
      frame "WRITE DO" {
        n73 = Variant To Data(type=T2 {"AO (real) 2"={"SCORTA 1"=0.0, "SCORTA 2"=0.0, "SCORTA 3"=0.0, "SCORTA 4"=0.0, "SCORTA 5"=0.0, "SCORTA 6"=0.0, "SCORTA 7"=0.0, "SCORTA 8"=0.0}, "statoAO_PLC out"={"Condensatori"=nan, "Scorta 1"=nan, "Scorta 2"=0.0}, "DO (bit)"={"Relè misura resistomat"=FALSE, "Misura res ramo 1"=FALSE, "Misura res ramo 2"=FALSE, "Misura res ramo 3"=FALSE, "Scelta banco 2"=FALSE, "Scala Torsiometro"=FALSE, "Ctrl torsiometro"=FALSE, "Select current mode"=FALSE, "Select Torque mode"=FALSE, "Select speed mode"=FALSE, "Watchdog"=FALSE, "Scorta"=FALSE, "Scorta 2"=FALSE, "Scorta 3"=FALSE, "Scorta 4"=FALSE, "Scorta 5"=FALSE, "Bench selection"=FALSE, "External alarm"=FALSE, "Enable external program"=FALSE, "Reset allarmi"=FALSE, "Start"=FALSE, "Stop"=FALSE, "Block"=FALSE, "Scorta 6"=FALSE}} ("USCITE PLC"), Variant=w185) -> (data=w180:T2)  [unwired: 1 in, 1 out]
        n74 = case shown="False" w182 {
          tunnel: w188 -> [w199 w235]
          tunnel: w187 -> [w198 w234]
          tunnel: w180 -> [w189 _]
          tunnel: [w193 w235] -> w184
          tunnel: [w192 w234] -> w183
          frame False {
            n75 = call "Mappa DO PLC_2.vi"("USCITE PLC 2"=w189) -> ("DO (DATABLOCK)"=w190:bool[], "DO (MERKER)"=w196:bool[])  [unwired: 9 in]
            "stato uscite DO" <- w196
            "DO (DATABLOCK)" <- w190
            n76 = local read "M BIT SCRITTURE"() -> (w197:cluster{"M":i16, "BIT":i16[]}[])
            n77 = for {
              tunnel: w197 -> [w232] mode=indexing
              shift-right: [w227] -> w195
              shift-left: w198 -> [w228]
              shift-right: [w225] -> _
              shift-left: w196 -> [w226]
              shift-right: [w229] -> w194
              shift-left: w199 -> [w230]
              # "scrivi per byte"
              n78 = Unbundle By Name(w232) -> ("M"=w231:i16)  [unwired: 1 out]
              n79 = Bundle By Name(cluster=T10 {"Read Length"=1, "Data Block #"=1, "S7_Add_Area"=131, "Start Address"=0, "S7_Transport_Size"=2, "S7_Function"=5} ("RW_CMD"), "Start Address"=w231) -> (w223:T10)
              n80 = Delete From Array(array=w226, length=8, index=0) -> (deleted portion=w221:bool[], array with subset deleted=w225:bool[])
              n81 = Boolean Array To Number(Boolean array=w221) -> (number=w219:u32)
              n82 = Build Array(w219) -> (w222:u32[])
              n83 = call "S7Com_WRT+READ(SubVI).vi"("Write_Data"=w222, "error in"=w228, "timeout ms (25000)"=5000, "RW_CMD"=w223, "connection ID in"=w230) -> ("error out"=w227:errorcluster, "connection ID out"=w229:refnum<k5>)  [unwired: 2 out]
            }
            n84 = local read "DB BIT SCRITTURE"() -> (w191:cluster{"DB":i16, "BIT":i16[], "DBoffset":i16}[])
            n85 = for {
              tunnel: w191 -> [w216] mode=indexing
              shift-right: [w211] -> w192
              shift-left: w195 -> [w212]
              shift-right: [w209] -> _
              shift-left: w190 -> [w210]
              shift-right: [w213] -> w193
              shift-left: w194 -> [w214]
              # "scrivi per byte"
              n86 = Unbundle By Name(w216) -> ("DB"=w215:i16, "DBoffset"=w200:i16)
              n87 = Bundle By Name(cluster=T10 {"Read Length"=1, "Data Block #"=1, "S7_Add_Area"=132, "Start Address"=0, "S7_Transport_Size"=2, "S7_Function"=5} ("RW_CMD"), "Data Block #"=w215, "Start Address"=w200) -> (w207:T10)
              n88 = Delete From Array(array=w210, length=8, index=0) -> (deleted portion=w205:bool[], array with subset deleted=w209:bool[])
              n89 = Boolean Array To Number(Boolean array=w205) -> (number=w203:u32)
              n90 = Build Array(w203) -> (w206:u32[])
              n91 = call "S7Com_WRT+READ(SubVI).vi"("Write_Data"=w206, "error in"=w212, "timeout ms (25000)"=5000, "RW_CMD"=w207, "connection ID in"=w214) -> ("error out"=w211:errorcluster, "connection ID out"=w213:refnum<k5>)  [unwired: 2 out]
            }
            "write do" <- w192
          }
          frame True {
            n92 = Wait (ms)(milliseconds to wait=u32 50) -> ()  [unwired: 1 out]
          }
        }
        n93 = Unbundle By Name(w180) -> ("DO (bit)"=w181:T4)
        n94 = Unbundle By Name(w178) -> ("AO (real) 2"=w176:T27, "statoAO_PLC out"=w177:T3)
        n95 = Bundle By Name(cluster=w178, "DO (bit)"=w181, "AO (real) 2"=w176, "statoAO_PLC out"=w177) -> (w179:T2)
        n96 = local write "USCITE PLC"(w179) -> ()
      }
      frame "STOP" {
        n97 = property on="stop" class="Bool (strict)"("Val(Sgnl)"=TRUE ("Value (Signaling)")) -> ()  [unwired: 2 in, 2 out]
        n98 = property on="stop" class="Bool (strict)"("Val(Sgnl)"=TRUE ("Value (Signaling)")) -> ()  [unwired: 2 in, 2 out]
      }
    }
    "Numeric" <- w26
  }
